vi "Seq File Menu Context Callback.vi"(4 "teststand-api out":refnum<class "teststand-api.lvclass">, 5 "Event Data":cluster{"menuHandle":i32, "x":i32, "y":i32}, 6 "Control Ref":refnum<k7>, 7 "Event Common Data":T1) -> ()   [LabVIEW 2014, in "teststand-api.lvlib" / "teststand-api.lvclass"]
uses:
  teststand-api.lvclass
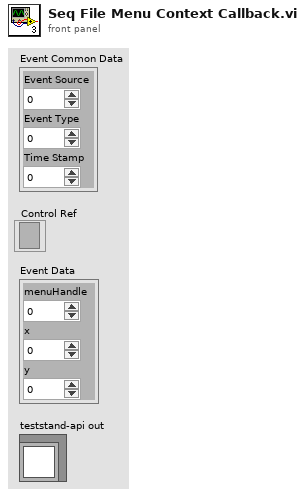
[diagram p1: front panel]
types:
  T1 = cluster{"Event Source":i32, "Event Type":u32, "Time Stamp":u32}
  T2 = typedef "teststand-api.lvlib/teststand-api.lvclass/Manager Controls Argument--cluster.ctl" = cluster{"App Manager":refnum<k7>, "Seq Manager":refnum<k7>, "Exec Manager":refnum<k7>}
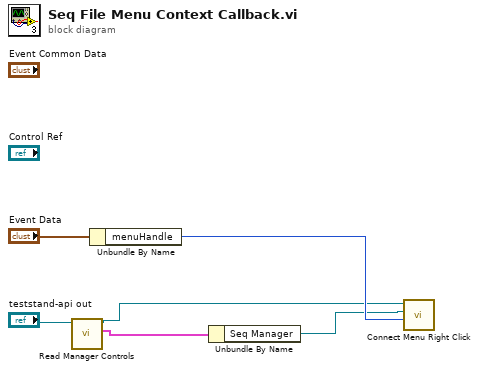
[diagram p0: block diagram]
diagram:
  n1 = call-dynamic "Read Manager Controls.vi"("teststand-api in"="teststand-api out") -> ("Manager Controls"=w1:T2, "teststand-api out"=w2:refnum<class "teststand-api.lvclass">)  [unwired: 8 in, 1 out]
  n2 = Unbundle By Name("Event Data") -> ("menuHandle"=w5:i32)
  n3 = Unbundle By Name(w1) -> ("Seq Manager"=w4:refnum<k7>)
  n4 = call "Connect Menu Right Click.vi"("menuHandle"=w5, "Manager Control"=w4, "teststand-api in"=w2) -> ()  [unwired: 7 in, 2 out]
